vi "reg.vi"(1 "Cluster":T2, 2 "C":bool, 3 "Reset":bool) -> (0 "output cluster":T1)   [LabVIEW 2012]
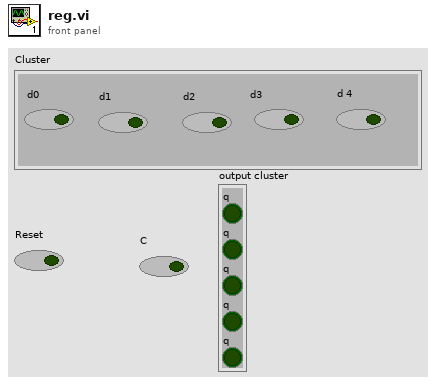
[diagram p1: front panel]
types:
  T1 = cluster{"q":bool, "q":bool, "q":bool, "q":bool, "q":bool}
  T2 = cluster{"d0":bool, "d1":bool, "d2":bool, "d3":bool, "d 4":bool}
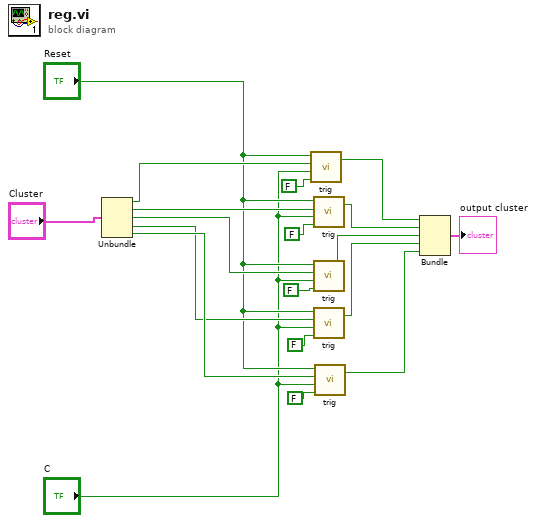
[diagram p0: block diagram]
diagram:
  n1 = Unbundle("Cluster") -> ("d0"=w14:bool, "d1"=w18:bool, "d2"=w17:bool, "d3"=w15:bool, "d 4"=w16:bool)
  n2 = call "trig.vi"("s"=FALSE, "c"="C", "d"=w14, "r"="Reset") -> ("q"=w6:bool)  [unwired: 1 out]
  n3 = call "trig.vi"("s"=FALSE ("Boolean"), "c"="C", "d"=w18, "r"="Reset") -> ("q"=w5:bool)  [unwired: 1 out]
  n4 = call "trig.vi"("s"=FALSE, "c"="C", "d"=w17, "r"="Reset") -> ("q"=w2:bool)  [unwired: 1 out]
  n5 = call "trig.vi"("s"=FALSE ("Boolean"), "c"="C", "d"=w15, "r"="Reset") -> ("q"=w3:bool)  [unwired: 1 out]
  n6 = call "trig.vi"("s"=FALSE, "c"="C", "d"=w16, "r"="Reset") -> ("q"=w4:bool)  [unwired: 1 out]
  n7 = Bundle("q"=w6, "q"=w5, "q"=w2, "q"=w3, "q"=w4) -> (→"output cluster":T1)  [unwired: 1 in]
